vi "poly_loop_timeout_value.vi"(1 "timeout (2k ms)":i32=2000, 2 "i (reset @ 0)":i32=1) -> (6 "remaining time":i32)   [LabVIEW 2015]
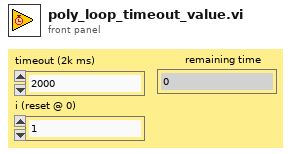
[diagram p1: front panel]
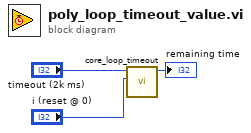
[diagram p0: block diagram]
diagram:
  n1 = call "core_loop_timeout.vi"("i (reset @ 0)"="i (reset @ 0)", "timeout (2k ms)"="timeout (2k ms)") -> ("remaining time"=→"remaining time":i32)  [unwired: 7 in, 1 out]
